vi "Close_uArm.vi"(8 "error in":errorcluster, 11 "VISA Refnum in":refnum<visa-resource-name>) -> (0 "error out":errorcluster)   [LabVIEW 2017]
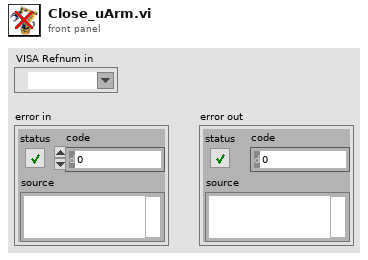
[diagram p1: front panel]
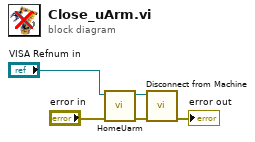
[diagram p0: block diagram]
diagram:
  n1 = call "HomeUarm.vi"("error in"="error in", "Machine In"="VISA Refnum in") -> ("error out"=w4:errorcluster, "Machine Out"=w1:refnum<visa-resource-name>)  [unwired: 8 in]
  n2 = call "Disconnect from Machine.vi"("error in"=w4, "Machine In"=w1) -> ("error out"=→"error out":errorcluster)  [unwired: 9 in]
